vi "Get Enclave.vi"(8 "error in (no error)":errorcluster, 11 "Tag in":refnum<class "Tag.lvclass">) -> (0 "error out":errorcluster, 2 "Enclave":refnum<class "Enclave.lvclass">, 3 "Tag out":refnum<class "Tag.lvclass">)   [LabVIEW 2022 SP3, in "Enclave.lvlib" / "Tag.lvclass"]
uses:
  Tag.lvclass
  Tag.lvclass/Tag.ctl
  Enclave/Enclave.lvclass
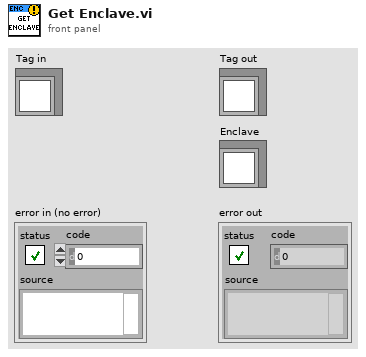
[diagram p1: front panel]
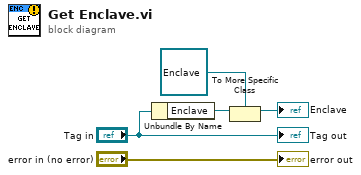
[diagram p0: block diagram]
diagram:
  n1 = Unbundle By Name("Tag in") -> ("Enclave"=w4:refnum<class>)
  n2 = To More Specific Class(target class=refnum<class "Enclave.lvclass"> refnum ("Enclave.lvlib:Enclave.lvclass"), reference=w4) -> (specific class reference=→"Enclave":refnum<class "Enclave.lvclass">)  [unwired: 1 in, 1 out]
  "error out" <- "error in (no error)"
  "Tag out" <- "Tag in"
